vi "14.Ultrasonic.vi"() -> ()   [LabVIEW 2017]
uses:
  <vilib>/myRIO/Instrument Drivers/Onboard IO/DIO/typedefs/DIO Reference.ctl
  <vilib>/myRIO/Common/Instrument Driver Framework/Utilities/typedefs/myRIO Generic Hardware Reference.ctl
  <vilib>/myRIO/Common/Instrument Driver Framework/Utilities/typedefs/Hardware Version Enum.ctl
  <vilib>/myRIO/Common/Instrument Driver Framework/Utilities/typedefs/myRIO v1.0 Reference.ctl
  <vilib>/myRIO/Common/Instrument Driver Framework/Utilities/typedefs/Generic FPGA Reference.ctl
  <vilib>/myRIO/Common/Instrument Driver Framework/myRIO v1.0/DIO/typedefs/DIO Channels List.ctl
  <vilib>/myRIO/Common/Instrument Driver Framework/myRIO v1.0/DIO/typedefs/DIO Channels Enum.ctl
  <vilib>/userdefined/High Color/nirio_resource_hc.ctl
  <vilib>/myRIO/Common/Instrument Driver Framework/myRIO v1.0/DIO/vis/myRIO v1.1 Open DIO.vi
  <vilib>/myRIO/Common/Instrument Driver Framework/Utilities/vis/Validate Channels.vi
  <vilib>/myRIO/Common/Instrument Driver Framework/myRIO v1.0/DIO/vis/myRIO v1.0 Reserve DIO.vi
  <vilib>/myRIO/Common/Instrument Driver Framework/myRIO v1.0/Resource Manager/vis/myRIO v1.0 Reserve Channel List.vi
  <vilib>/myRIO/Common/Instrument Driver Framework/myRIO v1.0/DIO/vis/myRIO v1.0 Build MUX Configuration DIO.vi
  <vilib>/myRIO/Common/Instrument Driver Framework/myRIO v1.0/Resource Manager/vis/myRIO v1.0 Reserve Channel.vi
  <vilib>/myRIO/Common/Instrument Driver Framework/myRIO v1.0/Resource Manager/vis/myRIO v1.0 Unreserve Channel.vi
  <vilib>/myRIO/Common/Instrument Driver Framework/myRIO v1.0/Resource Manager/vis/myRIO v1.0 Create Configuration List.vi
  <vilib>/myRIO/Common/Instrument Driver Framework/myRIO v1.0/Resource Manager/vis/myRIO v1.0 Build Mutex Name.vi
  <vilib>/Utility/VariantDataType/GetNumericInfo.vi
  <vilib>/Utility/error.llb/Error Cluster From Error Code.vi
  <vilib>/myRIO/Common/Instrument Driver Framework/myRIO v1.0/myRIO v1.1 Open.vi
  <vilib>/myRIO/Common/Instrument Driver Framework/Utilities/vis/IO Manager.vi
  <vilib>/myRIO/Common/Instrument Driver Framework/Utilities/vis/Configuration Manager.vi
  <vilib>/myRIO/Common/Instrument Driver Framework/myRIO v1.0/Resource Manager/vis/myRIO v1.0 Configure IO.vi
  <vilib>/myRIO/Common/Instrument Driver Framework/myRIO v1.0/myRIO v1.0 Close.vi
  <vilib>/myRIO/Common/Instrument Driver Framework/myRIO v1.0/DIO/vis/myRIO v1.0 Write DIO.vi
  <vilib>/myRIO/Common/Instrument Driver Framework/myRIO v1.0/DIO/vis/myRIO v1.0 Read DIO.vi
  <vilib>/myRIO/Instrument Drivers/Onboard IO/DIO/vis/myRIO DIO Open.xnode
  <vilib>/myRIO/Instrument Drivers/Onboard IO/DIO/DIO.lvlib
panel:
  out "波形图表":dbl(graph)
  in  "当前温度":dbl
  in  "停止":bool
  out "超声波测距":dbl
  in  "error in (no error)":errorcluster
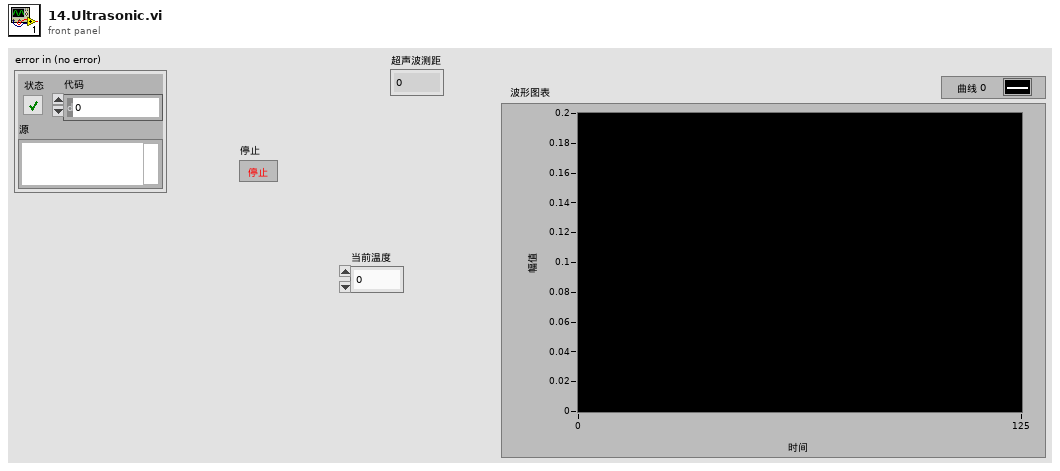
[diagram p1: front panel]
types:
  T1 = typedef "nirio_resource_hc.ctl" = tag
  T2 = typedef "Hardware Version Enum.ctl" = enum16{"Unknown", "myRIO-1900", "myRIO-1950", "roboRIO", "NI ELVIS RIO CM"}
  T3 = typedef "DIO.lvlib/DIO Reference.ctl" = cluster{"myRIO Reference":T4, "DIO Channels List":T7}
  T4 = typedef "myRIO Generic Hardware Reference.ctl" = cluster{"myRIO Model":T2, "myRIO Hardware Reference":T5}
  T5 = typedef "myRIO v1.0 Reference.ctl" = cluster{"Generic FPGA Reference":T6, "Allow multiple opens":bool}
  T6 = typedef "Generic FPGA Reference.ctl" = refnum<k20>
  T7 = typedef "DIO Channels List.ctl" = T8[]
  T8 = typedef "DIO Channels Enum.ctl" = enum16{"Not Connected", "C/DIO0", "C/DIO1", "C/DIO2", "C/DIO3", "C/DIO4", "C/DIO5", "C/DIO6", "C/DIO7", "A/DIO0", "A/DIO1", "A/DIO2", "A/DIO3", "A/DIO4", "A/DIO5", "A/DIO6", "A/DIO7", "A/DIO8", "A/DIO9", "A/DIO10", "A/DIO11", "A/DIO12", "A/DIO13", "A/DIO14", "A/DIO15", "B/DIO0", "B/DIO1", "B/DIO2", "B/DIO3", "B/DIO4", "B/DIO5", "B/DIO6", "B/DIO7", "B/DIO8", "B/DIO9", "B/DIO10", "B/DIO11", "B/DIO12", "B/DIO13", "B/DIO14", "B/DIO15", "LED0", "LED1", "LED2", "LED3", "Button0", "DIO/DIO0", "DIO/DIO1", "DIO/DIO2", "DIO/DIO3", "DIO/DIO4", "DIO/DIO5", "DIO/DIO6", "DIO/DIO7", "DIO/DIO8", "DIO/DIO9", "SPI/CS0", "SPI/CS1", "SPI/CS2", "SPI/CS3", "LED RADIO (Green)", "LED RADIO (Red)", "LED COMM (Green)", "LED COMM (Red)", "LED MODE (Green)", "LED MODE (Red)"}
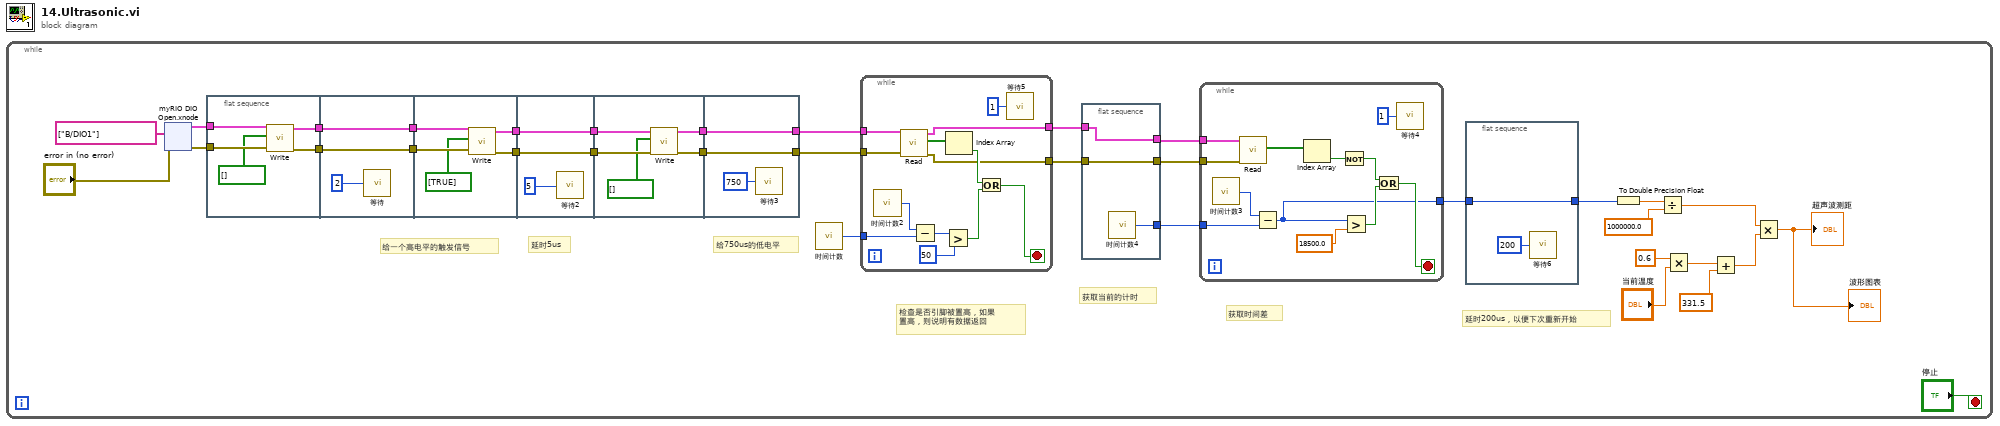
[diagram p0: block diagram]
diagram:
  n1 = while {
    stop <- "停止" stop-if-true
    # "延时200us，以便下次重新开始"
    # "获取时间差"
    # "获取当前的计时"
    # "检查是否引脚被置高，如果\n置高，则说明有数据返回"
    # "给750us的低电平"
    # "延时5us"
    # "给一个高电平的触发信号"
    n2 = xnode "myRIO DIO Open.xnode"("error in (no error)"="error in (no error)", "Channel Names"=tag[] ["B/DIO1"]) -> ("error out"=w31:errorcluster, "DIO Ref Out"=w32:T3)  [unwired: 1 in]
    n3 = flat-sequence {
      tunnel: w32 -> [w69]
      tunnel: w31 -> [w68]
      tunnel: [w66] -> w29
      tunnel: [w65] -> w27
      tunnel: [w71] -> w30
      tunnel: w29 -> [w71]
      tunnel: [w70] -> w28
      tunnel: w27 -> [w70]
      tunnel: w30 -> [w77]
      tunnel: w28 -> [w76]
      tunnel: [w74] -> w26
      tunnel: [w73] -> w25
      tunnel: w26 -> [w78]
      tunnel: w25 -> [w79]
      tunnel: [w79] -> w24
      tunnel: [w78] -> w23
      tunnel: w24 -> [w85]
      tunnel: w23 -> [w84]
      tunnel: [w82] -> w22
      tunnel: [w81] -> w21
      tunnel: [w87] -> w20
      tunnel: w22 -> [w87]
      tunnel: [w86] -> w19
      tunnel: w21 -> [w86]
      frame #0 {
        n4 = call <vilib>:"Write.vi"("error in (no error)"=w68, "Values"=bool[] [], "DIO Ref In"=w69) -> ("error out"=w65:errorcluster, "DIO Ref Out"=w66:T3)  [unwired: 6 in]
      }
      frame #1 {
        n5 = call "等待"("Count(uSec)"=u32 2) -> ()  [unwired: 1 out]
      }
      frame #2 {
        n6 = call <vilib>:"Write.vi"("error in (no error)"=w76, "Values"=bool[] [TRUE], "DIO Ref In"=w77) -> ("error out"=w73:errorcluster, "DIO Ref Out"=w74:T3)  [unwired: 6 in]
      }
      frame #3 {
        n7 = call "等待2"("Count(uSec)"=u32 5) -> ()  [unwired: 1 out]
      }
      frame #4 {
        n8 = call <vilib>:"Write.vi"("error in (no error)"=w85, "Values"=bool[] [], "DIO Ref In"=w84) -> ("error out"=w81:errorcluster, "DIO Ref Out"=w82:T3)  [unwired: 6 in]
      }
      frame #5 {
        n9 = call "等待3"("Count(uSec)"=u32 750 ("Count(mSec)")) -> ()  [unwired: 1 out]
      }
    }
    n10 = call "时间计数"() -> ("Tick Count(uSec)"=w18:u32)
    n11 = while {
      tunnel: w20 -> [w64]
      tunnel: w19 -> [w63]
      tunnel: w18 -> [w62]
      tunnel: [w54] -> w17
      tunnel: [w53] -> w16
      stop <- w55 stop-if-true
      n12 = call "时间计数2"() -> ("Tick Count(uSec)"=w61:u32)
      n13 = call <vilib>:"Read.vi"("error in (no error)"=w63, "DIO Ref In"=w64) -> ("error out"=w53:errorcluster, "Values"=w58:bool[], "DIO Ref Out"=w54:T3)  [unwired: 7 in]
      n14 = Subtract(x=w61, y=w62) -> (x-y=w60:u32)
      n15 = Greater?(x=w60, y=u32 50) -> (0:w56:bool)
      n16 = Index Array(array=w58) -> (element=w57:bool)  [unwired: 1 in]
      n17 = Or(x=w57, y=w56) -> (x .or. y?=w55:bool)
      n18 = call "等待5"("Count(uSec)"=u32 1) -> ()  [unwired: 1 out]
    }
    n19 = flat-sequence {
      tunnel: w17 -> [w38]
      tunnel: w16 -> [w39]
      tunnel: [w39] -> w14
      tunnel: [w38] -> w15
      tunnel: [w37] -> w13
      frame #0 {
        n20 = call "时间计数4"() -> ("Tick Count(uSec)"=w37:u32)
      }
    }
    n21 = while {
      tunnel: w15 -> [w51]
      tunnel: w14 -> [w50]
      tunnel: w13 -> [w42]
      tunnel: [w40] -> w9
      stop <- w44 stop-if-true
      n22 = call "时间计数3"() -> ("Tick Count(uSec)"=w43:u32)
      n23 = call <vilib>:"Read.vi"("error in (no error)"=w50, "DIO Ref In"=w51) -> ("Values"=w49:bool[])  [unwired: 7 in, 2 out]
      n24 = Subtract(x=w43, y=w42) -> (x-y=w40:u32)
      n25 = Index Array(array=w49) -> (element=w48:bool)  [unwired: 1 in]
      n26 = Not(x=w48) -> (.not. x?=w47:bool)
      n27 = Greater?(x=w40, y=18500.0) -> (0:w46:bool)
      n28 = Or(x=w47, y=w46) -> (x .or. y?=w44:bool)
      n29 = call "等待4"("Count(uSec)"=u32 1) -> ()  [unwired: 1 out]
    }
    n30 = flat-sequence {
      tunnel: [w35] -> w8
      tunnel: w9 -> [w35]
      frame #0 {
        n31 = call "等待6"("Count(uSec)"=u32 200) -> ()  [unwired: 1 out]
      }
    }
    n32 = To Double Precision Float(number=w8) -> (double precision float=w12:dbl)
    n33 = Divide(x=w12, y=1000000.0) -> (x/y=w2:dbl)
    n34 = Multiply(x=0.6, y="当前温度") -> (x*y=w4:dbl)
    n35 = Add(x=w4, y=331.5) -> (x+y=w3:dbl)
    n36 = Multiply(x=w2, y=w3) -> (x*y=→"超声波测距" →"波形图表":dbl)
  }
